vi "RT Close LabVIEW.vi"(8 "error in (no error)":errorcluster) -> (0 "error out":errorcluster)   [LabVIEW 2020]
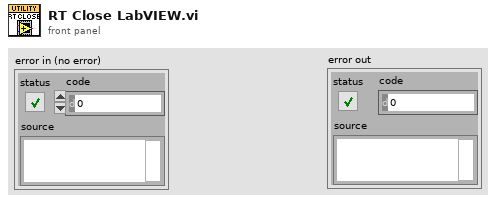
[diagram p1: front panel]
types:
  T1 = enum32{"invalid app kind", "Development System", "Run Time System", "Student Edition", "Embedded LabVIEW", "Evaluation", "Custom"}
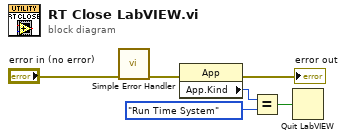
[diagram p0: block diagram]
diagram:
  n1 = call <vilib>:"Simple Error Handler.vi"("error in (no error)"="error in (no error)") -> ("error out"=w1:errorcluster)  [unwired: 4 in, 4 out]
  n2 = property class="App"(error in=w1) -> (error out=→"error out":errorcluster, "App.Kind"=w4:T1)  [unwired: 1 in, 1 out]
  n3 = Equal?(x=w4, y=T1."Run Time System" ("Application:Kind")) -> (x = y?=w3:bool)
  n4 = Quit LabVIEW(quit? (T)=w3) -> ()
